vi "sub-Language global.vi"() -> ()   [LabVIEW 2011]
panel:
  out "languages":T1(array[cluster])
  out "menu items":string[](array[string])
  out "selected":i32
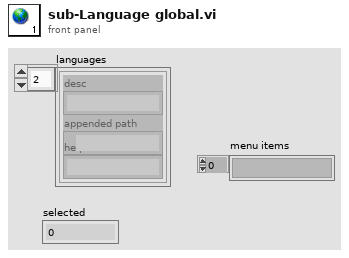
[diagram p1: front panel]
types:
  T1 = cluster{"desc":string, "appended path":path, "help dir":string}[]
diagram:
